vi "main_.vi"() -> ()   [LabVIEW 2018]
uses:
  <vilib>/Analysis/4window.llb/windowTd.ctl
  <vilib>/DAQmx/read.llb/DAQmx Read (Analog Wfm 1Chan NSamp).vi
  <vilib>/Analysis/5stat.llb/RMS (DBL).vi
  <vilib>/DAQmx/create/channels.llb/DAQmx Create Channel (AI-Voltage-Basic).vi
  <vilib>/DAQmx/configure/timing.llb/DAQmx Timing (Sample Clock).vi
  <vilib>/DAQmx/miscellaneous.llb/DAQmx Fill In Error Info.vi
  <vilib>/measure/maspectr.llb/FFT Spectrum (Mag-Phase) for 1 Chan.vi
  <vilib>/measure/matone.llb/Harmonic Distortion Analyzer 1 Chan.vi
  <vilib>/Analysis/NI_AALPro.lvlib
  <vilib>/measure/NI_MAPro.lvlib
  <vilib>/measure/NI_MABase.lvlib
panel:
  in  "Amplituda":dbl
  in  "Šum":dbl
  out "RMS filtrovaného signálu":dbl(graph)
  out "RMS original signálu":dbl(graph)
  out "RMS value filtrovaneho signalu [V]":dbl format="%0.2f"
  out "Amplitudově frekvenční spektrum (50kS/s)":cluster{"f0":dbl, "df":dbl, "magnitude":dbl[]}(graph)
  out "FFT (50kS/s)":cluster{"f0":dbl, "df":dbl, "magnitude":dbl[]}(graph)
  out "Amplitudově frekvenční spektrum (5kS/s)":cluster{"f0":dbl, "df":dbl, "magnitude":dbl[]}(graph)
  out "Základní harmonická":dbl format="%.2p"
  out "FFT (5kS/s)":cluster{"f0":dbl, "df":dbl, "magnitude":dbl[]}(graph)
  out "- Počet vzroků po decimaci":i32
  out "- Počet vzorků před decimací":i32
  out "Filtr + decimace (5kS/s)":waveform(dbl)(graph)
  out "Čtení dat uložených na disku":waveform(dbl)[](graph)
  in  "PrecistSoubor":bool
  in  "Který soubor chcete otevřít?":path
  out "Časové razítko souboru:":string
  out "- List všech uložených souborů":i32(listbox)
  out "Trigr":bool
  out "Nejnovější pokles":waveform(dbl)[](graph)
  out "RMS value [V]":dbl format="%0.2f"
  in  "Trigr. podminka [V]":dbl
  in  "Směr průchodu":bool
  in  "Prah detekce [V]":dbl
  out "Sledovaný signál":waveform(dbl)(graph)
  in  "stop":bool
  # "- Musí být menší než amplituda signálu (doporučuje se použít 0)"
  # "-  Určuje velikost při kterém se bude trgrovat uložení do souoru."
  # "- Určuje, jakým směrem bude program určovat průchod nulou.\n(Doporučuje se použít směr průchodů \"dolů\")."
  # "- RMS hodnota je určena aktuálnímu měření."
  # "- Červená křivka je křivka PŘED poklesem.\n- Bílá křivak je u které bylo RMS vyhodnoceno \npod trigrovací úroveň.\n\nPOZN.:\nPokud se zobrazí pouze jeden průběh, znamená to, že triggr byl zachycen při prvním běhu aplikace a\nnení předchozí průběh na zobrazení. Tudíž se zobrazí pouze průběh s poklesem."
  # "Využívá se pouze při simulaci signálu"
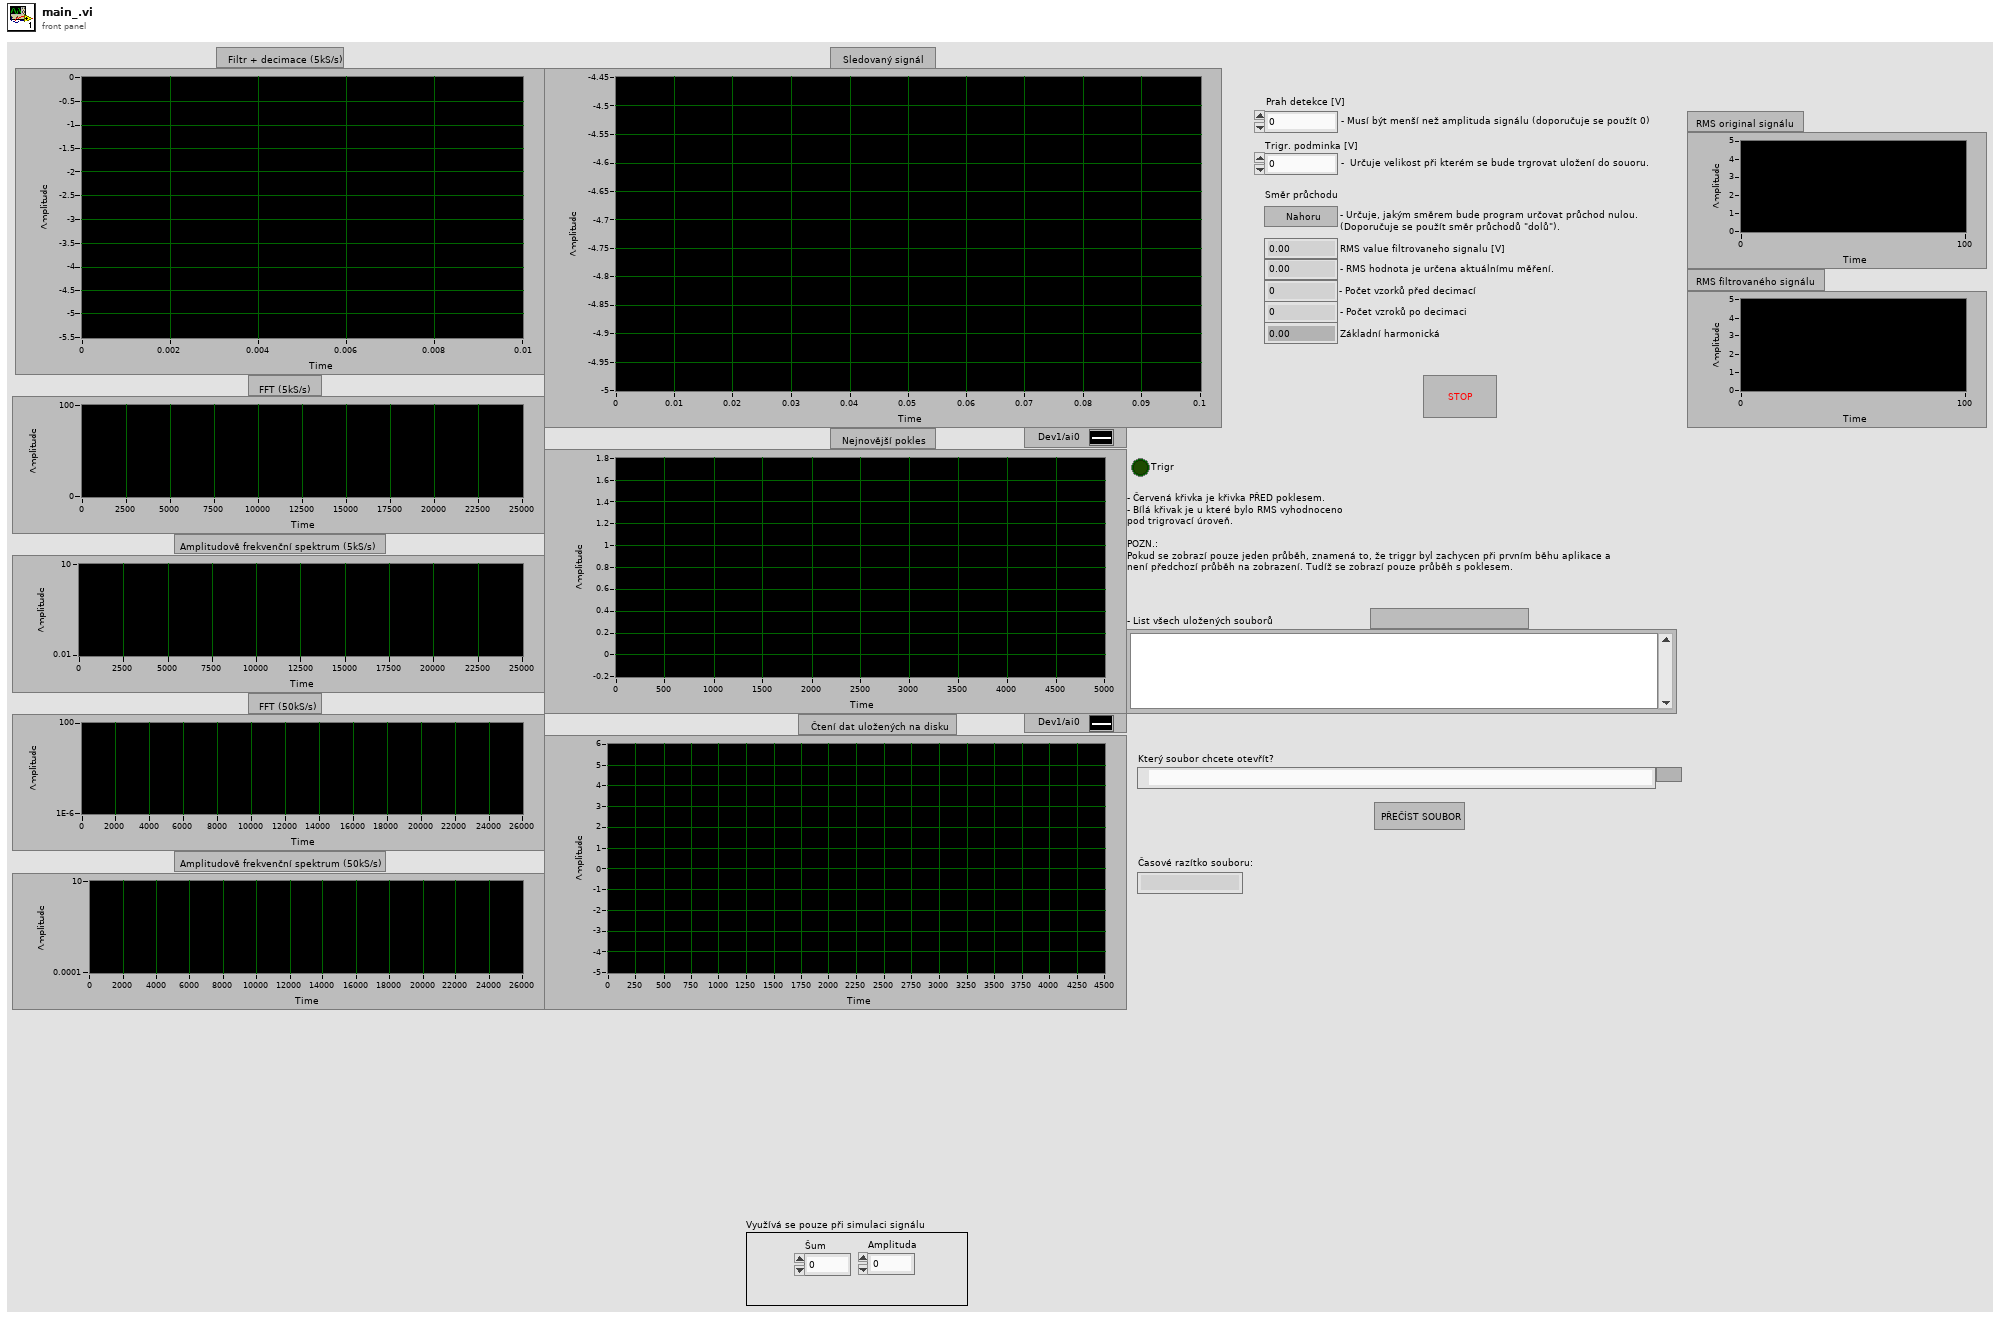
[diagram p1: front panel]
types:
  T1 = cluster{"dB On (F)":bool, "unwrap phase (F)":bool, "convert to degree (F)":bool}
  T2 = enum16{"Sine Wave", "Triangle Wave", "Square Wave", "Sawtooth Wave"}
  T3 = typedef "NI_AALPro.lvlib/windowTd.ctl" = u32
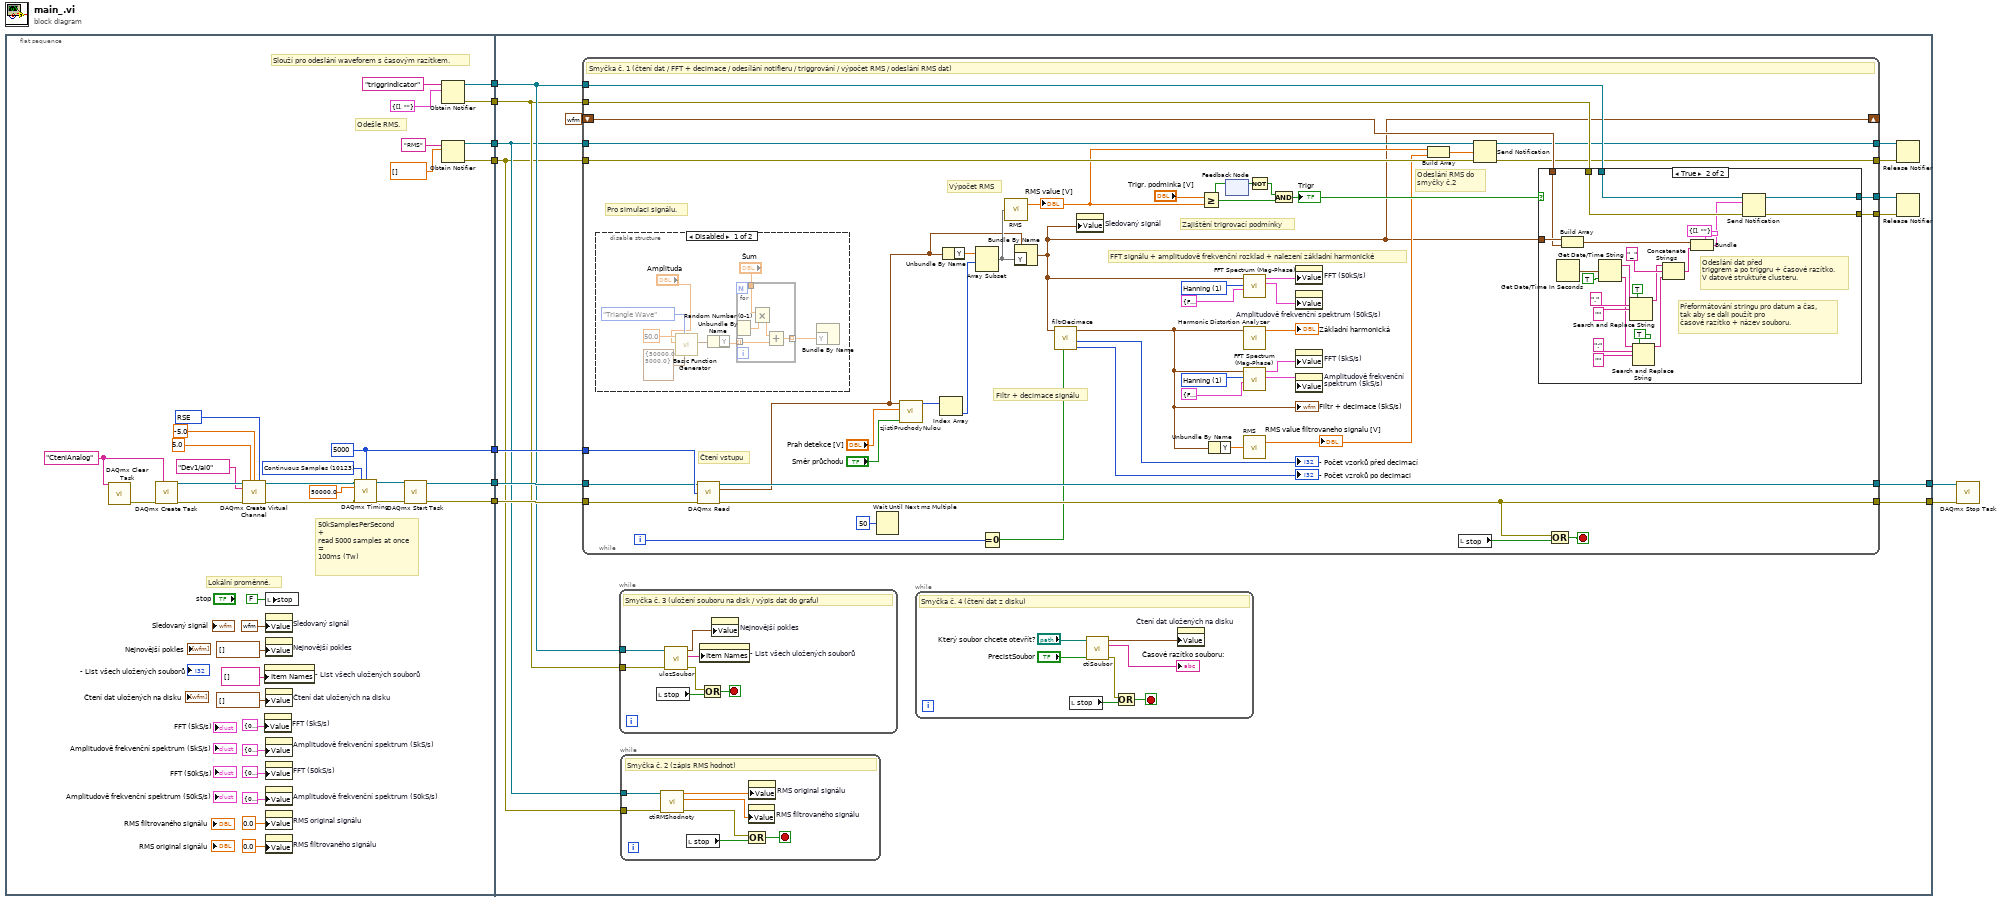
[diagram p0: block diagram]
diagram:
  n1 = flat-sequence {
    tunnel: [w31] -> w9
    tunnel: [w30] -> w8
    tunnel: [w29] -> w7
    tunnel: [w25] -> w4
    tunnel: [w24] -> w3
    tunnel: [w13] -> w2
    tunnel: [w12] -> w1
    tunnel: w9 -> [w59]
    tunnel: w8 -> [w58]
    tunnel: w7 -> [w57]
    tunnel: [w56] -> w6
    tunnel: [w55] -> w5
    tunnel: w4 -> [w53]
    tunnel: w3 -> [w52]
    tunnel: w2 -> [w47]
    tunnel: w1 -> [w46]
    frame #0 {
      w38 = "CteniAnalog" ("new task name")
      w37 = 10123 items=["Finite Samples"=10178, "Continuous Samples"=10123, "Hardware Timed Single Point"=12522] ("sample mode")
      w31 = 5000 ("number of samples per channel")
      w33 = 10083 items=["Default"=-1, "RSE"=10083, "NRSE"=10078, "Differential"=10106, "Pseudodifferential"=12529] ("input terminal configuration")
      # "Odešle RMS."
      # "Slouží pro odeslání waveforem s časovým razítkem."
      # "Lokální proměnné."
      # "50kSamplesPerSecond\n+\nread 5000 samples at once\n=\n100ms (Tw)"
      n2 = call <vilib>:"DAQmx Clear Task.vi"("task in"=w38) -> ("error out"=w42:errorcluster)  [unwired: 14 in]
      n3 = call <vilib>:"DAQmx Create Task.vi"("new task name"=w38, "error in"=w42) -> ("task out"=w44:refnum<k21>, "error out"=w43:errorcluster)  [unwired: 12 in]
      n4 = call-poly <vilib>:"DAQmx Create Virtual Channel.vi"("task in"=w44, "maximum value"=5.0, "minimum value"=-5.0, "input terminal configuration"=w33, "physical channels"=tag "Dev1/ai0", "error in"=w43) -> ("task out"=w45:refnum<k21>, "error out"=w39:errorcluster)  [unwired: 8 in]
      n5 = property on="- List všech uložených souborů" class="LstBox (strict)"("Item Names"=string[] []) -> ()  [unwired: 2 in, 2 out]
      n6 = property on="FFT (5kS/s)" class="WFGraph (strict)"("Value"=cluster{"f0":dbl, "df":dbl, "magnitude":dbl[]} {"f0"=0.0, "df"=0.0, "magnitude"=[]} ("FFT")) -> ()  [unwired: 2 in, 2 out]
      n7 = local write "stop"(FALSE) -> ()
      n8 = property on="Sledovaný signál" class="WFGraph (strict)"("Value"=waveform(dbl) {"t0"=timestamp(0 s since 1904-01-01), "dt"=1.0, "Y"=[]} ("Waveform Graph")) -> ()  [unwired: 2 in, 2 out]
      n9 = property on="Nejnovější pokles" class="WFGraph (strict)"("Value"=waveform(dbl)[] []) -> ()  [unwired: 2 in, 2 out]
      n10 = property on="Čtení dat uložených na disku" class="WFGraph (strict)"("Value"=waveform(dbl)[] [] ("Čtení dat uložených na disku")) -> ()  [unwired: 2 in, 2 out]
      n11 = property on="Amplitudově frekvenční spektrum (5kS/s)" class="WFGraph (strict)"("Value"=cluster{"f0":dbl, "df":dbl, "magnitude":dbl[]} {"f0"=0.0, "df"=0.0, "magnitude"=[]} ("Amplitudově frekvenční spektrum")) -> ()  [unwired: 2 in, 2 out]
      n12 = property on="FFT (50kS/s)" class="WFGraph (strict)"("Value"=cluster{"f0":dbl, "df":dbl, "magnitude":dbl[]} {"f0"=0.0, "df"=0.0, "magnitude"=[]} ("FFT")) -> ()  [unwired: 2 in, 2 out]
      n13 = property on="Amplitudově frekvenční spektrum (50kS/s)" class="WFGraph (strict)"("Value"=cluster{"f0":dbl, "df":dbl, "magnitude":dbl[]} {"f0"=0.0, "df"=0.0, "magnitude"=[]} ("Amplitudově frekvenční spektrum")) -> ()  [unwired: 2 in, 2 out]
      n14 = property on="RMS original signálu" class="WFChart (strict)"("Value"=0.0 ("RMS original signálu")) -> ()  [unwired: 2 in, 2 out]
      n15 = property on="RMS filtrovaného signálu" class="WFChart (strict)"("Value"=0.0 ("RMS original signálu")) -> ()  [unwired: 2 in, 2 out]
      n16 = call-poly <vilib>:"DAQmx Timing.vi"("task/channels in"=w45, "sample mode"=w37, "samples per channel"=w31, "rate"=50000.0, "error in"=w39) -> ("task out"=w40:refnum<k21>, "error out"=w41:errorcluster)  [unwired: 9 in]
      n17 = call <vilib>:"DAQmx Start Task.vi"("task/channels in"=w40, "error in"=w41) -> ("task out"=w30:refnum<k21>, "error out"=w29:errorcluster)  [unwired: 12 in]
      n18 = Obtain Notifier(name (unnamed)="triggrIndicator", notification data type=cluster{waveform(dbl)[], string} {[], ""}) -> (notifier out=w25:refnum<notifier>, error out=w24:errorcluster)  [unwired: 2 in, 1 out]
      n19 = Obtain Notifier(name (unnamed)="RMS", notification data type=dbl[] []) -> (notifier out=w13:refnum<notifier>, error out=w12:errorcluster)  [unwired: 2 in, 1 out]
    }
    frame #1 {
      n20 = while {
        tunnel: w59 -> [w128]
        tunnel: w58 -> [w127]
        tunnel: w57 -> [w126]
        tunnel: [w125] -> w56
        tunnel: [w123] -> w55
        shift-right: [w90] -> _
        shift-left: waveform(dbl) {"t0"=timestamp(0 s since 1904-01-01), "dt"=1.0, "Y"=[]} -> [w101]
        tunnel: w53 -> [w113]
        tunnel: w52 -> [w112]
        tunnel: [w111] -> w51
        tunnel: [w110] -> w50
        tunnel: w47 -> [w100]
        tunnel: w46 -> [w99]
        tunnel: [w95] -> w49
        tunnel: [w94] -> w48
        i -> [w109]
        stop <- w122 stop-if-true
        w83 = T3 1 items=["Rectangle"=0, "Hanning"=1, "Hamming"=2, "Blackman-Harris"=3, "Exact Blackman"=4, "Blackman"=5, "Flat Top"=6, "4 Term B-Harris "=7, "7 Term B-Harris"=8, "Low Sidelobe"=9, "Blackman Nuttall"=11, "Triangle"=30, "Bartlett-Hanning"=31, "Bohman"=32, "Parzen"=33, "Welch"=34, "Kaiser"=60, "Dolph-Chebyshev"=61, "Gaussian"=62] ("window")
        w108 = T3 1 items=["Rectangle"=0, "Hanning"=1, "Hamming"=2, "Blackman-Harris"=3, "Exact Blackman"=4, "Blackman"=5, "Flat Top"=6, "4 Term B-Harris "=7, "7 Term B-Harris"=8, "Low Sidelobe"=9, "Blackman Nuttall"=11, "Triangle"=30, "Bartlett-Hanning"=31, "Bohman"=32, "Parzen"=33, "Welch"=34, "Kaiser"=60, "Dolph-Chebyshev"=61, "Gaussian"=62] ("window")
        # "Pro simulaci signálu."
        # "FFT signálu + amplitudově frekvenční rozklad + nalezení základní harmonické"
        # "Filtr + decimace signálu"
        # "Odeslání RMS do \nsmyčky č.2"
        # "Čtení vstupu"
        # "Zajištění trigrovací podmínky"
        # "Výpočet RMS"
        # "Smyčka č. 1 (čtení dat / FFT + decimace / odesílání notifieru / triggrování / výpočet RMS / odeslání RMS dat)"
        n21 = disable-structure shown="Disabled" {
          frame Disabled {
            n22 = call <vilib>:"Basic Function Generator.vi"("sampling info"=cluster{"Fs":dbl, "#s":dbl} {"Fs"=50000.0, "#s"=5000.0}, "signal type"=T2."Triangle Wave", "amplitude"="Amplituda", "frequency"=50.0) -> ("signal out"=w130:waveform(dbl))  [unwired: 5 in, 2 out]
            n23 = Unbundle By Name(w130) -> ("Y"=w133:dbl[])
            n24 = for {
              tunnel: w133 -> [w140] mode=indexing
              tunnel: [w141] -> w129 mode=indexing
              tunnel: "Šum" -> [w139]
              n25 = Random Number (0-1)() -> (number: 0 to 1=w137:dbl)
              n26 = Multiply(x=w139, y=w137) -> (x*y=w138:dbl)
              n27 = Add(x=w138, y=w140) -> (x+y=w141:dbl)
            }
            n28 = Bundle By Name("Y"=w129) -> ()  [unwired: 1 in, 1 out]
          }
          frame Enabled {
          }
        }
        n29 = call-poly <vilib>:"DAQmx Read.vi"("task/channels in"=w127, "number of samples per channel"=w128, "error in"=w126) -> ("task out"=w125:refnum<k21>, "data"=w81:waveform(dbl), "error out"=w123:errorcluster)  [unwired: 10 in]
        n30 = Wait Until Next ms Multiple(millisecond multiple=u32 50) -> ()  [unwired: 1 out]
        n31 = call "zjistiPruchodyNulou.vi"("smerPruchodu"="Směr průchodu", "prahDetekce"="Prah detekce [V]", "vstupniSignal"=w81) -> ("vsechnyPruchody"=w91:i32[])  [unwired: 8 in]
        n32 = Index Array(array=w91) -> (element=w120:i32)  [unwired: 1 in]
        n33 = Unbundle By Name(w81) -> ("Y"=w82:dbl[])
        n34 = Array Subset(array=w82, index=w120) -> (w119:dbl[])  [unwired: 1 in]
        n35 = Equal To 0?(x=w109) -> (x = 0?=w89:bool)
        n36 = call-poly <vilib>:"RMS.vi"("X"=w119) -> ("rms value"=w98:dbl)  [unwired: 1 out]
        "RMS value [V]" <- w98
        n37 = Bundle By Name(cluster=w81, "Y"=w119) -> (w90:waveform(dbl))
        n38 = call "filtrDecimace.vi"("inicializace"=w89, "vstupniWaveform"=w90) -> ("vzorkyPoDecimaci"=→"- Počet vzroků po decimaci":i32, "vzorkyPredDecimaci"=→"- Počet vzorků před decimací":i32, "vystupniWaveform"=w87:waveform(dbl))  [unwired: 7 in]
        "Filtr + decimace (5kS/s)" <- w87
        n39 = property on="Sledovaný signál" class="WFGraph (strict)"("Value"=w90) -> ()  [unwired: 2 in, 2 out]
        n40 = Greater Or Equal?(x="Trigr. podminka [V]", y=w98) -> (x >= y?=w116:bool)
        n41 = Unbundle By Name(w87) -> ("Y"=w88:dbl[])
        n42 = feedback-in #1(w116) -> ()
        n43 = feedback #1() -> (w115:bool)  [unwired: 1 in]
        n44 = call-poly <vilib>:"FFT Spectrum (Mag-Phase).vi"("view"=T1 {"dB On (F)"=FALSE, "unwrap phase (F)"=FALSE, "convert to degree (F)"=FALSE}, "window"=w83, "time signal"=w90) -> ("phase"=w102:cluster{"f0":dbl, "df":dbl, "phase":dbl[]}, "magnitude"=w103:cluster{"f0":dbl, "df":dbl, "magnitude":dbl[]})  [unwired: 4 in, 3 out]
        n45 = call-poly <vilib>:"Harmonic Distortion Analyzer.vi"("signal in"=w87) -> ("detected fundamental frequency"=→"Základní harmonická":dbl)  [unwired: 5 in, 5 out]
        n46 = call-poly <vilib>:"FFT Spectrum (Mag-Phase).vi"("view"=T1 {"dB On (F)"=FALSE, "unwrap phase (F)"=FALSE, "convert to degree (F)"=FALSE}, "window"=w108, "time signal"=w87) -> ("phase"=w104:cluster{"f0":dbl, "df":dbl, "phase":dbl[]}, "magnitude"=w105:cluster{"f0":dbl, "df":dbl, "magnitude":dbl[]})  [unwired: 4 in, 3 out]
        n47 = call-poly <vilib>:"RMS.vi"("X"=w88) -> ("rms value"=w96:dbl)  [unwired: 1 out]
        "RMS value filtrovaneho signalu [V]" <- w96
        n48 = Not(x=w115) -> (.not. x?=w117:bool)
        n49 = And(x=w117, y=w116) -> (x .and. y?=w114:bool)
        "Trigr" <- w114
        n50 = property on="FFT (50kS/s)" class="WFGraph (strict)"("Value"=w103) -> ()  [unwired: 2 in, 2 out]
        n51 = property on="Amplitudově frekvenční spektrum (50kS/s)" class="WFGraph (strict)"("Value"=w102) -> ()  [unwired: 2 in, 2 out]
        n52 = property on="FFT (5kS/s)" class="WFGraph (strict)"("Value"=w105) -> ()  [unwired: 2 in, 2 out]
        n53 = property on="Amplitudově frekvenční spektrum (5kS/s)" class="WFGraph (strict)"("Value"=w104) -> ()  [unwired: 2 in, 2 out]
        n54 = Build Array(w98, w96) -> (w97:dbl[])
        n55 = local read "stop"() -> (w124:bool)
        n56 = Send Notification(notification=w97, notifier=w100, error in (no error)=w99) -> (notifier out=w95:refnum<notifier>, error out=w94:errorcluster)
        n57 = case shown="True" w114 {
          tunnel: w101 -> [_ w165]
          tunnel: w90 -> [_ w166]
          tunnel: w113 -> [w143 w164]
          tunnel: w112 -> [w142 w163]
          tunnel: [w143 w162] -> w111
          tunnel: [w142 w161] -> w110
          frame False {
          }
          frame True {
            # "Odeslání dat před \ntriggrem a po triggru + časové razítko.\nV datové struktuře clusteru."
            # "Přeformátování stringu pro datum a čas, \ntak aby se dali použít pro \nčasové razítko + název souboru."
            n58 = Get Date/Time In Seconds() -> (seconds since 1Jan1904=w157:timestamp)
            n59 = Build Array(w166, w165) -> (w159:waveform(dbl)[])
            n60 = Get Date/Time String(seconds (now)=w157, want seconds? (F)=TRUE) -> (date string=w152:string, time string=w145:string)  [unwired: 1 in]
            n61 = Search and Replace String(replace all?=TRUE ("replace all? (F)"), input string=w152, search string=".", replace string="" ("replace string (\"\")")) -> (result string=w149:string)  [unwired: 4 in, 3 out]
            n62 = Search and Replace String(replace all?=TRUE ("replace all? (F)"), input string=w145, search string=":", replace string="" ("replace string (\"\")")) -> (result string=w146:string)  [unwired: 4 in, 3 out]
            n63 = Concatenate Strings(w149, "_", w146) -> (w155:string)
            n64 = Bundle(cluster=cluster{waveform(dbl)[], string} {[], ""}, w159, w155) -> (w158:cluster{waveform(dbl)[], string})
            n65 = Send Notification(notification=w158, notifier=w164, error in (no error)=w163) -> (notifier out=w162:refnum<notifier>, error out=w161:errorcluster)
          }
        }
        n66 = Compound Arithmetic op=OR(w123, w124) -> (w122:bool)
      }
      n67 = while {
        tunnel: w53 -> [w75]
        tunnel: w52 -> [w76]
        stop <- w79 stop-if-true
        # "Smyčka č. 3 (uložení souboru na disk / výpis dat do grafu)"
        n68 = local read "stop"() -> (w80:bool)
        n69 = call "ulozSoubor.vi"("vstupniError"=w76, "vstupniNotifier"=w75) -> ("vystupniError"=w77:errorcluster, "vystupniString"=w78:string[], "vystupWaveforma"=w74:waveform(dbl)[])  [unwired: 7 in]
        n70 = property on="- List všech uložených souborů" class="LstBox (strict)"("Item Names"=w78) -> ()  [unwired: 2 in, 2 out]
        n71 = Compound Arithmetic op=OR(w77, w80) -> (w79:bool)
        n72 = property on="Nejnovější pokles" class="WFGraph (strict)"("Value"=w74) -> ()  [unwired: 2 in, 2 out]
      }
      n73 = while {
        tunnel: w47 -> [w64]
        tunnel: w46 -> [w63]
        stop <- w65 stop-if-true
        # "Smyčka č. 2 (zápis RMS hodnot)"
        n74 = call "ctiRMShodnoty.vi"("vstupniError"=w63, "vstupniNotifier"=w64) -> ("vystupniError"=w60:errorcluster, "RMS filtrovaného signálu"=w61:dbl, "RMS original signálu"=w62:dbl)  [unwired: 7 in]
        n75 = local read "stop"() -> (w66:bool)
        n76 = property on="RMS filtrovaného signálu" class="WFChart (strict)"("Value"=w61) -> ()  [unwired: 2 in, 2 out]
        n77 = property on="RMS original signálu" class="WFChart (strict)"("Value"=w62) -> ()  [unwired: 2 in, 2 out]
        n78 = Compound Arithmetic op=OR(w60, w66) -> (w65:bool)
      }
      n79 = while {
        stop <- w72 stop-if-true
        # "Smyčka č. 4 (čtení dat z disku)"
        n80 = local read "stop"() -> (w73:bool)
        n81 = call "ctiSoubor.vi"("PrecistSoubor"="PrecistSoubor", "Který soubor chcete otevřít?"="Který soubor chcete otevřít?") -> ("vystupniError"=w71:errorcluster, "Časové razítko souboru:"=→"Časové razítko souboru:":string, "data"=w69:waveform(dbl)[])  [unwired: 7 in]
        n82 = Compound Arithmetic op=OR(w71, w73) -> (w72:bool)
        n83 = property on="Čtení dat uložených na disku" class="WFGraph (strict)"("Value"=w69) -> ()  [unwired: 2 in, 2 out]
      }
      n84 = Release Notifier(notifier=w49, error in (no error)=w48) -> ()  [unwired: 1 in, 3 out]
      n85 = Release Notifier(notifier=w51, error in (no error)=w50) -> ()  [unwired: 1 in, 3 out]
    }
  }
  n86 = call <vilib>:"DAQmx Stop Task.vi"("task/channels in"=w6, "error in"=w5) -> ()  [unwired: 12 in, 2 out]
